vi "CmdConsole._Test Run and Wait.vi"() -> ()   [LabVIEW 2018]
uses:
  CmdConsole.lvclass
panel:
  out "Duration":dbl
  in  "Timeout(s)":dbl=1.0 format="%#_13g"
  out "error out":errorcluster
  out "Rtn Code":i32
  out "StdError":string
  out "Stdout":string
  in  "Args":string="--capture c:\\MTE\\Capture.png 110"
  in  "App":path=path "C:/Users/eddiek/Dropbox/Valve MTE SW/MTE Testers/HMD/Hmd Control and Status App/Camera/vrcamera_console.exe"
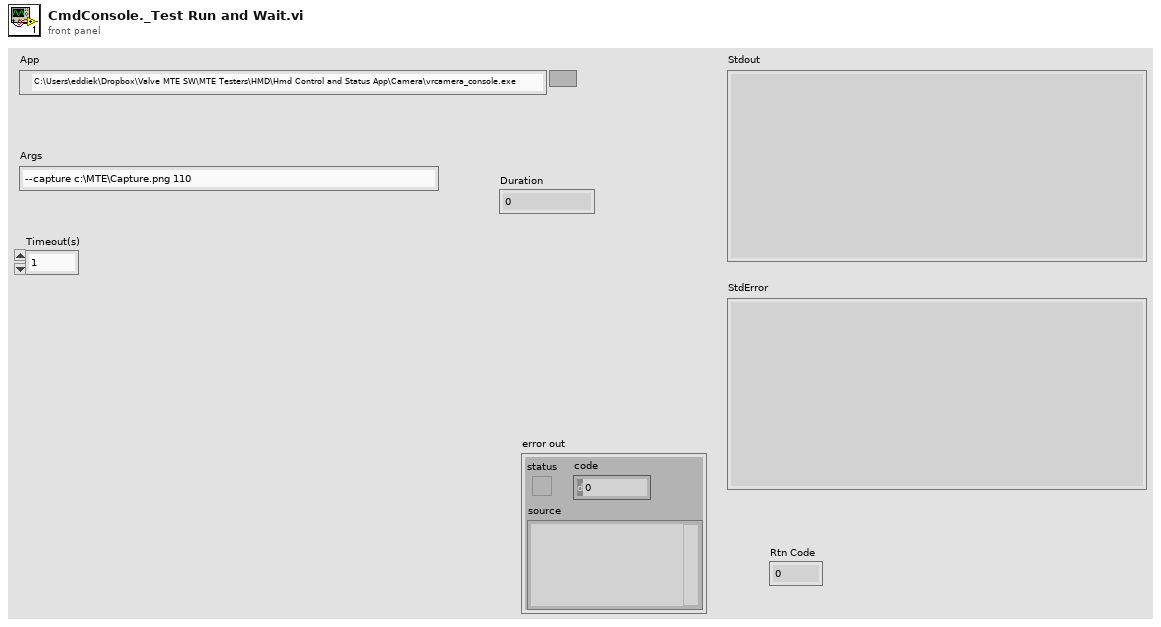
[diagram p1: front panel]
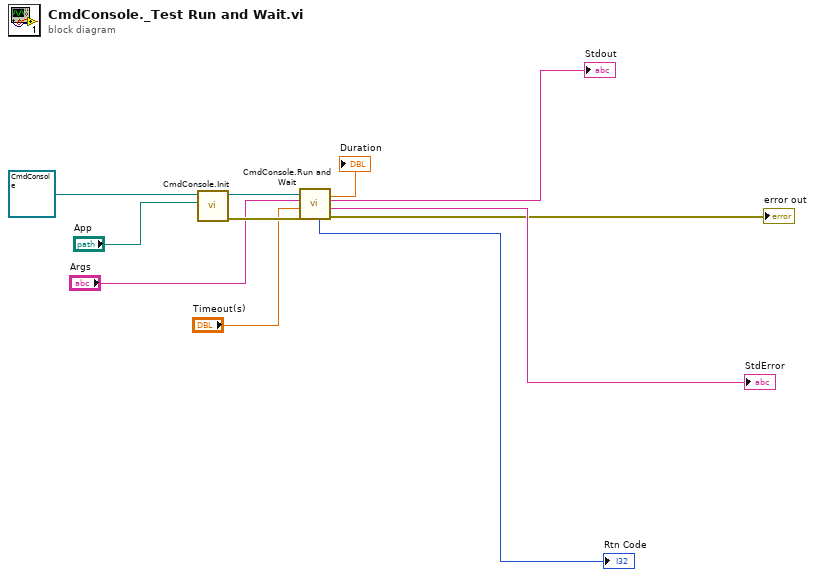
[diagram p0: block diagram]
diagram:
  n1 = call "CmdConsole.Init.vi"("App"="App", "CmdConsole in"=refnum<class "CmdConsole.lvclass"> refnum ("CmdConsole.lvclass")) -> ("error out"=w4:errorcluster, "CmdConsole out"=w11:refnum<class "CmdConsole.lvclass">)  [unwired: 8 in]
  n2 = call "CmdConsole.Run and Wait.vi"("error in (no error)"=w4, "Timeout(s)"="Timeout(s)", "Args"="Args", "CmdConsole in"=w11) -> ("error out"=→"error out":errorcluster, "Std Error"=→"StdError":string, "Std Out"=→"Stdout":string, "RtnCode"=→"Rtn Code":i32, "Duration"=→"Duration":dbl)  [unwired: 2 in, 1 out]
